vi "AAA Hacker A150-12.vi"() -> ()   [LabVIEW 2020]
uses:
  <instrlib>/Gantner Instruments/Ethernet/Gantner-Instruments HighSpeedPort.llb/e.gate Protocol Type.ctl
  <vilib>/Instr/_visa.llb/VISA Configure Serial Port (Instr).vi
  <vilib>/Utility/file.llb/Write Delimited Spreadsheet (string).vi
panel:
  out "Value":dbl[](graph)
  out "Elapsed Time":string
  out "?":dbl[](array[slide]) scale=0.0..1000.0
  out "Temperature 2":dbl[](array[slide]) caption="Thermocouple 1" scale=20.0..50.0
  out "error out 2":errorcluster
  in  "?":bool
  out "Random Number":dbl(knob) scale=0.0..180.0
  out "error out":errorcluster
  in  "START":bool
  out "PWM Feedback":string
  in  "PWM Value":string
  # "Hacker A150-12  -  Motor control"
  # "Temperatures"
  # "READ ME"
  # "The minimum value to get the motor started is 25. \n\nWhen done with testing, put in a value of 0 BEFORE HITTING THE STOP BUTTON.\n\nData is saved in MotorTestBench (excell sheet)\n\n\nSeperate Arduino should be used for Atmospheric Conditions"
  # "Torque"
  # "Power Supply"
  # "Atmospheric\nConditions"
  # "Voltage"
  # "Thrust"
  # "Current"
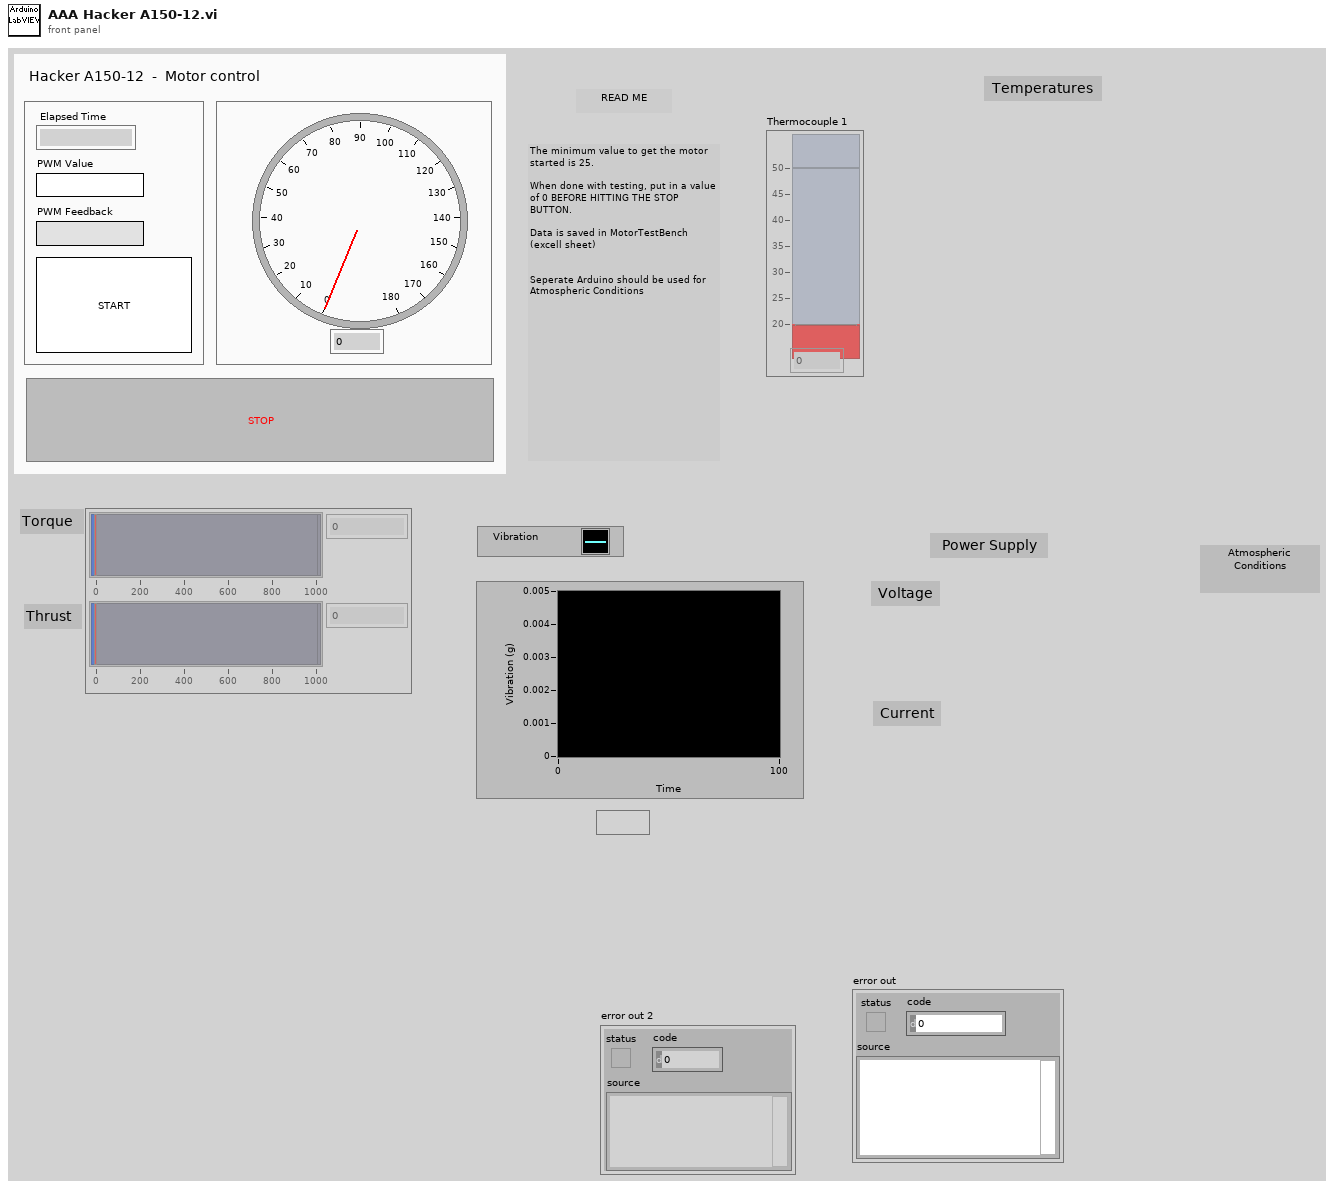
[diagram p1: front panel]
types:
  T1 = typedef "e.gate Protocol Type.ctl" = enum16{"ASCII", "HighspeedPort Online", "HighspeedPort Buffer (giutility.DLL) ", "PostProcessBuffer (giutility.DLL)", "HighspeedPort Online (giutility.DLL)", "Decode UDBF File (giutility.DLL)"}
  T2 = typedef "e.gate Configuration.ctl" = cluster{"connection ID":refnum<k5>, "IPAddress":string, "BufferIndex":i32, "StateMessage":string, "StateCode":i8, "HeaderSize":i32, "BufferSize":i32, "IsBigEndian":i32, "Version":i32, "ChannelCount":i32, "FrameLength":i32, "StartTime":dbl, "dActTimeToSecondFactor":dbl, "StartTimeToDayFactor":dbl, "BufferFillRate":dbl, "SampleRate":dbl, "ChannelData":T3[], "DecodeTimeFormat":string, "SummaryPath":string, "WithCheckSum":i32, "dActTimeDataType":T4, "MaxWriteCount":i32, "MaxReadCount":i32, "TempOffsetRead":i32, "TempLengthRead":i32, "Protocol":T1, "IsSupported":i32, "InputAccessList":i32[], "OutputAccessList":i32[], "DataSource":enum16{"CircleBuffer", "test.con Logger", "test.con Archive"}, "Modules":T5[], "DLL-Handle":T6}
  T3 = typedef "e.gate Channel Data.ctl" = cluster{"VariableName":string, "DataDirection":string, "DataType":string, "DataTypeIndex":T4, "Precision":i16, "FieldLengtht":i16, "ByteCount":i32, "Format":string, "Unit":string, "InputAccessOffset":i32, "OutputAccessOffset":i16, "InputAccessIndex":i16, "OutputAccessIndex":i16, "VarType":string}
  T4 = typedef "e.gate Data Type.ctl" = enum16{"NO", "BOOL", "SINT8", "USINT8", "SINT16", "USINT16", "SINT32", "USINT32", "FLOAT", "SET8", "SET16", "SET32", "DOUBLE", "SINT64", "USINT64", "SET64"}
  T5 = typedef "e.gate Module  Data.ctl" = cluster{"Type":string, "Location":string, "VariablesCount":i16, "UartIndex":i16, "Address":i16, "SystemOffset":i16}
  T6 = typedef "e.gateHSP_DLLhandle.ctl" = cluster{"clientInstance":i32, "connectionInstance":i32, "Is32Bit":bool, "DLL Path":path}
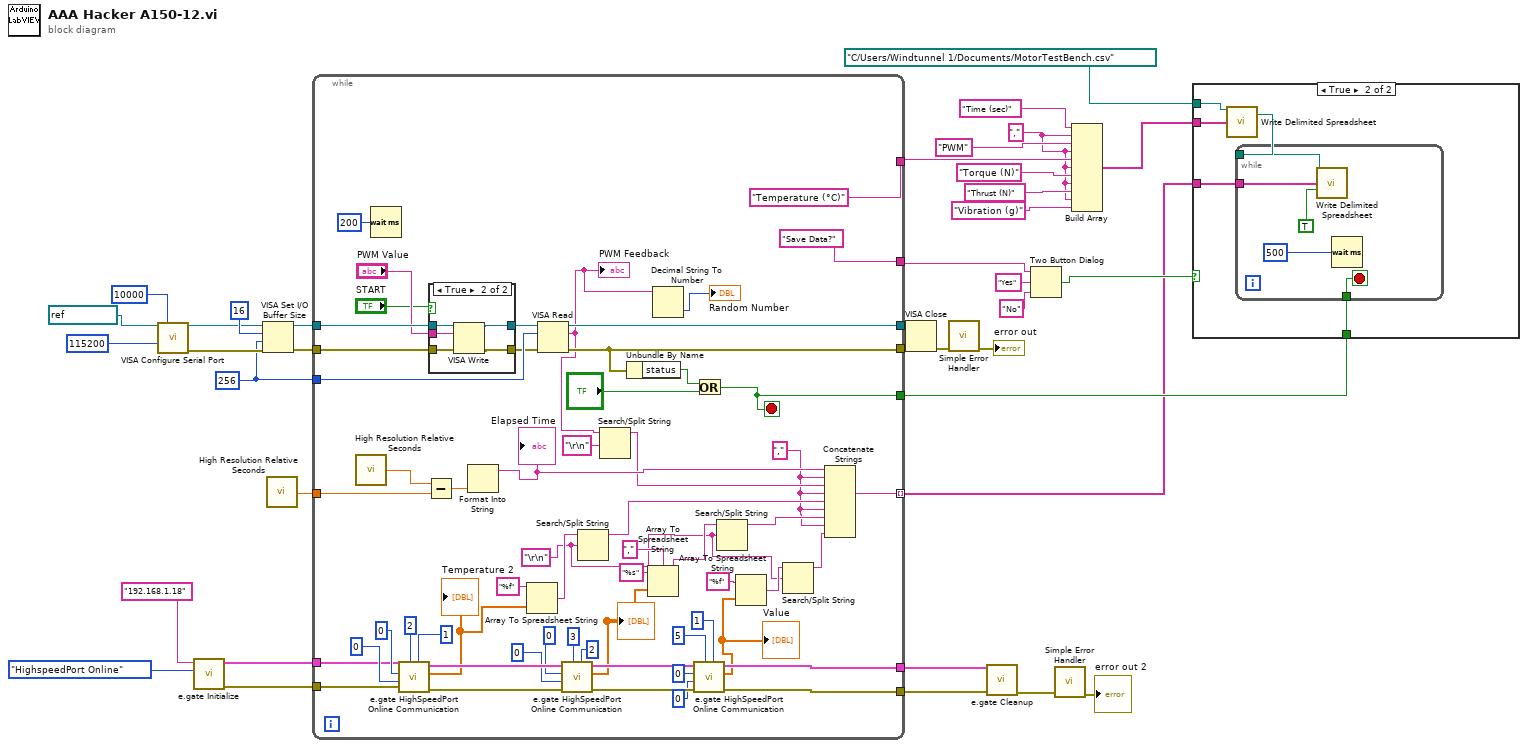
[diagram p0: block diagram]
diagram:
  w2 = "," ("element")
  w25 = u32 256 ("buffer size")
  n1 = call-poly "VISA Configure Serial Port"("VISA resource name"=refnum<visa-resource-name> "COM5", "timeout (10sec)"=u32 10000, "baud rate (9600)"=u32 115200) -> ("VISA resource name out"=w34:refnum<visa-resource-name>, "error out"=w33:errorcluster)  [unwired: 11 in]
  n2 = call <instrlib>:"e.gate Initialize.vi"("Protocol"=e.gate_Protocol_Type."HighspeedPort Online", "IP Address"="192.168.1.18") -> ("error out"=w19:errorcluster, "e.gate Configuration"=w20:T2)  [unwired: 8 in]
  n3 = VISA Set I/O Buffer Size(VISA resource name=w34, mask (16)=u16 16 ("I/O Receive\nBuffer mask"), size (4096)=w25, error in (no error)=w33) -> (VISA resource name out=w32:refnum<visa-resource-name>, error out=w31:errorcluster)
  n4 = call <vilib>:"High Resolution Relative Seconds.vi"() -> ("relative seconds"=w8:dbl)
  n5 = while {
    tunnel: w32 -> [w94]
    tunnel: w31 -> [w93]
    tunnel: [w95] -> w37
    tunnel: [w86] -> w36
    tunnel: w25 -> [w96]
    tunnel: w20 -> [w73]
    tunnel: w19 -> [w72]
    tunnel: [w52] -> w18
    tunnel: [w53] -> w17
    tunnel: ["Save Data?" ("message")] -> w12
    tunnel: [w70] -> w11
    tunnel: ["Temperature (°C)" ("element")] -> w10
    tunnel: w8 -> [w66]
    tunnel: [w47] -> w9 mode=indexing
    stop <- w70 stop-if-true
    w40 = "\r\n" ("search string/char (-)")
    w38 = "," ("string")
    n6 = call <vilib>:"High Resolution Relative Seconds.vi"() -> ("relative seconds"=w67:dbl)
    n7 = Wait (ms)(milliseconds to wait=u32 200) -> ()  [unwired: 1 out]
    n8 = call <instrlib>:"e.gate HighSpeedPort Online Communication.vi"("ReadCount"=1, "ReadIndex"=2, "error in (no error)"=w72, "WriteCount"=0, "WriteIndex"=0, "e.gate Configuration In"=w73) -> ("error out"=w78:errorcluster, "Value"=w68:dbl[], "e.gate Configuration Out"=w79:T2)  [unwired: 3 in]
    "Temperature 2" <- w68
    n9 = Subtract(x=w67, y=w66) -> (x-y=w65:dbl)
    n10 = case shown="True" "START" {
      tunnel: w94 -> [w98 w103]
      tunnel: w93 -> [w97 w102]
      tunnel: [w98 w101] -> w92
      tunnel: [w97 w100] -> w91
      tunnel: "PWM Value" -> [_ w99]
      frame False {
      }
      frame True {
        n11 = VISA Write(VISA resource name=w103, write buffer=w99, error in (no error)=w102) -> (VISA resource name out=w101:refnum<visa-resource-name>, error out=w100:errorcluster)  [unwired: 1 out]
      }
    }
    n12 = Format Into String(w65) -> (resulting string=w60:string)  [unwired: 3 in, 1 out]
    "Elapsed Time" <- w60
    n13 = Array To Spreadsheet String(array=w68, 3:"%f" ("format string")) -> (spreadsheet string=w61:string)  [unwired: 1 in]
    n14 = VISA Read(VISA resource name=w92, byte count=w96, error in (no error)=w91) -> (VISA resource name out=w95:refnum<visa-resource-name>, read buffer=w57:string, error out=w86:errorcluster)  [unwired: 1 out]
    "PWM Feedback" <- w57
    n15 = call <instrlib>:"e.gate HighSpeedPort Online Communication.vi"("ReadCount"=2, "ReadIndex"=3, "error in (no error)"=w78, "WriteCount"=0, "WriteIndex"=0, "e.gate Configuration In"=w79) -> ("error out"=w54:errorcluster, "Value"=w55:dbl[], "e.gate Configuration Out"=w56:T2)  [unwired: 3 in]
    "?" <- w55
    n16 = Search/Split String(string=w61, search string/char (-)=w40) -> (substring before match=w45:string)  [unwired: 1 in, 2 out]
    n17 = Search/Split String(string=w57, search string/char (-)="\r\n") -> (substring before match=w59:string)  [unwired: 1 in, 2 out]
    n18 = Unbundle By Name(w86) -> ("status"=w85:bool)
    n19 = Array To Spreadsheet String(delimiter (Tab)=",", array=w55, 3:"%s" ("format string")) -> (spreadsheet string=w46:string)
    n20 = Decimal String To Number(string=w57) -> (number=→"Random Number":i32)  [unwired: 2 in, 1 out]
    n21 = call <instrlib>:"e.gate HighSpeedPort Online Communication.vi"("ReadCount"=1, "ReadIndex"=5, "error in (no error)"=w54, "WriteCount"=0, "WriteIndex"=0, "e.gate Configuration In"=w56) -> ("error out"=w53:errorcluster, "Value"=w43:dbl[], "e.gate Configuration Out"=w52:T2)  [unwired: 3 in]
    "Value" <- w43
    n22 = Or(x=w85, y="?") -> (x .or. y?=w70:bool)
    n23 = Search/Split String(string=w46, search string/char (-)=w40) -> (substring before match=w44:string)  [unwired: 1 in, 2 out]
    n24 = Array To Spreadsheet String(array=w43, 3:"%f" ("format string")) -> (spreadsheet string=w41:string)  [unwired: 1 in]
    n25 = Search/Split String(string=w41, search string/char (-)=w40) -> (substring before match=w39:string)  [unwired: 1 in, 2 out]
    n26 = Concatenate Strings(w60, w38, w59, w38, w45, w38, w44, w38, w39) -> (w47:string)
  }
  n27 = VISA Close(VISA resource name=w37, error in (no error)=w36) -> (error out=w30:errorcluster)
  n28 = call <vilib>:"Simple Error Handler.vi"("error in (no error)"=w30) -> ("error out"=→"error out":errorcluster)  [unwired: 4 in, 4 out]
  n29 = call <instrlib>:"e.gate Cleanup.vi"("error in (no error)"=w17, "e.gate Configuration"=w18) -> ("error out"=w24:errorcluster)  [unwired: 9 in]
  n30 = Two Button Dialog(message=w12, 1:"No" ("F button name (\"Cancel\")"), 2:"Yes" ("T button name (\"OK\")")) -> (T button?=w15:bool)
  n31 = call <vilib>:"Simple Error Handler.vi"("error in (no error)"=w24) -> ("error out"=→"error out 2":errorcluster)  [unwired: 4 in, 4 out]
  n32 = Build Array("Time (sec)" ("element"), w2, "PWM" ("element"), w2, w10, w2, "Torque (N)" ("element"), w2, "Thrust (N)" ("element"), w2, "Vibration (g)" ("element")) -> (w16:string[])
  n33 = case shown="True" w15 {
    tunnel: w16 -> [_ w107]
    tunnel: w11 -> [_ w106]
    tunnel: w9 -> [_ w105]
    tunnel: path "C:/Users/Windtunnel 1/Documents/MotorTestBench.csv" ("file path (dialog if empty) 2") -> [_ w104]
    frame False {
    }
    frame True {
      n34 = call-poly <vilib>:"Write Delimited Spreadsheet.vi"("file path (dialog if empty)"=w104, "1D data"=w107) -> ("new file path (Not A Path if cancelled)"=w108:path)  [unwired: 12 in, 1 out]
      n35 = while {
        tunnel: w108 -> [w113]
        tunnel: w106 -> [w110]
        tunnel: w105 -> [w109]
        stop <- w110 stop-if-true
        n36 = call-poly <vilib>:"Write Delimited Spreadsheet.vi"("file path (dialog if empty)"=w113, "1D data"=w109, "append to file? (new file:F)"=TRUE) -> ()  [unwired: 11 in, 2 out]
        n37 = Wait (ms)(milliseconds to wait=u32 500) -> ()  [unwired: 1 out]
      }
    }
  }
